vi "Rational Resample (single channel, CDB).vi"(5 "anti-aliasing?":bool=TRUE, 6 "FIR filter specifications":T1={"alias rejection (dB)"=120.0, "normalized bandwidth"=0.4536} {"normalized bandwidth" format="%.4f"; "alias rejection (dB)" format="%.2f"}, 7 "reset":bool, 8 "error in (no error)":errorcluster, 9 "resample factor":cluster{"interpolation":i32, "decimation":i32}={"interpolation"=1, "decimation"=1}, 10 "start index":i32, 11 "X":cdb[](array[numeric])) -> (0 "error out":errorcluster, 2 "t0":dbl, 3 "Y":cdb[](array[numeric]))   [LabVIEW 2014, in "NI_AALPro.lvlib"]
doc: "Resamples the input signal <B>X</B> by interpolating <B>X</B>, passing the interpolated signal through an FIR filter, and decimating the filtered signal. Wire data to the <B>X</B> input to determine the polymorphic instance to use or manually select the instance."
uses:
  NI_AALPro.lvlib
  lvanlys.dll
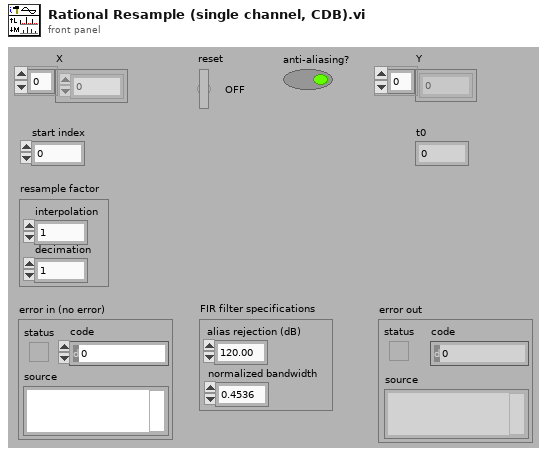
[diagram p1: front panel]
types:
  T1 = cluster{"alias rejection (dB)":dbl, "normalized bandwidth":dbl}
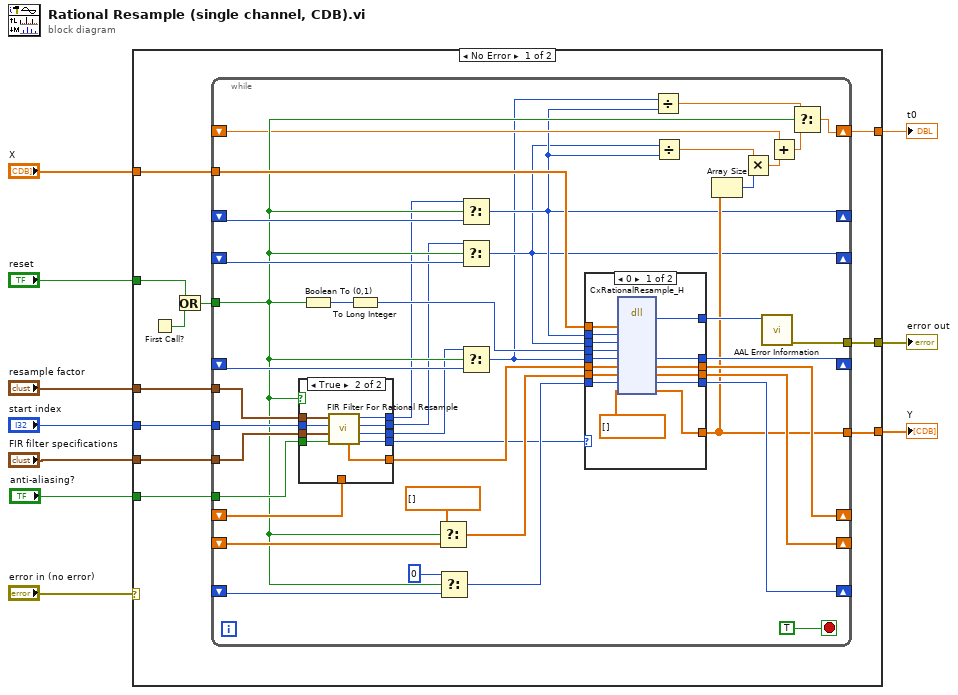
[diagram p0: block diagram]
diagram:
  n1 = case shown="No Error" "error in (no error)" {
    selector: "error in (no error)" -> [_ w89]
    tunnel: "X" -> [w21 _]
    tunnel: "FIR filter specifications" -> [w20 _]
    tunnel: "start index" -> [w19 _]
    tunnel: [w18 w89] -> w7
    tunnel: "resample factor" -> [w17 _]
    tunnel: [w16 _] -> w5
    tunnel: "anti-aliasing?" -> [w15 _]
    tunnel: [w14 _] -> w2
    tunnel: "reset" -> [w11 _]
    frame No Error {
      n2 = First Call?() -> (First Call?: T/F=w13:bool)
      n3 = Or(x=w11, y=w13) -> (x .or. y?=w12:bool)
      n4 = while {
        tunnel: w21 -> [w62]
        shift-right: [w25] -> _
        shift-left: _ -> [w60]
        tunnel: w12 -> [w36]
        shift-right: [w24] -> _
        shift-left: _ -> [w59]
        shift-right: [w43] -> _
        shift-left: _ -> [w56]
        shift-right: [w44] -> _
        shift-left: _ -> [w54]
        shift-right: [w50] -> _
        shift-left: _ -> [w51]
        shift-right: [w47] -> _
        shift-left: _ -> [w46]
        tunnel: w20 -> [w49]
        tunnel: w19 -> [w45]
        tunnel: [w41] -> w18
        tunnel: w17 -> [w40]
        tunnel: [w33] -> w16
        tunnel: w15 -> [w37]
        shift-right: [w34] -> w14
        shift-left: _ -> [w27]
        stop <- TRUE stop-if-true
        n5 = case shown="True" w36 {
          tunnel: [w79 w82] -> w48
          tunnel: w49 -> [_ w83]
          tunnel: w46 -> [w79 _]
          tunnel: [_ w88] -> w32
          tunnel: [_ w87] -> w31
          tunnel: w45 -> [_ w84]
          tunnel: [_ w86] -> w22
          tunnel: w40 -> [_ w85]
          tunnel: [_ w81] -> w39
          tunnel: w37 -> [_ w80]
          frame False {
          }
          frame True {
            n6 = call "FIR Filter For Rational Resample.vi"("anti-aliasing?"=w80, "FIR filter specifications"=w83, "start index"=w84, "resample factor"=w85) -> ("error"=w81:i32, "start index out"=w86:i32, "decimation"=w87:i32, "interpolation out"=w88:i32, "filter coefficients"=w82:dbl[])  [unwired: 3 in]
          }
        }
        n7 = Boolean To (0,1)(Boolean=w36) -> (0, 1=w58:i16)
        n8 = To Long Integer(number=w58) -> (32bit integer=w57:i32)
        n9 = Select(t=cdb[] [] ("yH"), s=w36, f=w56) -> (s? t:f=w52:cdb[])
        n10 = Select(t=0, s=w36, f=w54) -> (s? t:f=w53:i32)
        n11 = Select(t=w32, s=w36, f=w60) -> (s? t:f=w25:i32)
        n12 = Select(t=w31, s=w36, f=w59) -> (s? t:f=w24:i32)
        n13 = Select(t=w22, s=w36, f=w51) -> (s? t:f=w23:i32)
        n14 = case shown="0" w39 {
          selector: w39 -> [_ w78]
          tunnel: w62 -> [w77 _]
          tunnel: w25 -> [w76 _]
          tunnel: w24 -> [w75 _]
          tunnel: w57 -> [w74 _]
          tunnel: w53 -> [w73 _]
          tunnel: w52 -> [w66 _]
          tunnel: w23 -> [w72 _]
          tunnel: [w71 _] -> w50
          tunnel: w48 -> [w70 _]
          tunnel: [w69 _] -> w47
          tunnel: [w68 _] -> w44
          tunnel: [w65 _] -> w43
          tunnel: [w67 w78] -> w42
          tunnel: [w63 _] -> w33
          frame 0 {
            n15 = dll-call lib="C:/Program Files (x86)/National Instruments/LabVIEW 2014/resource/lvanlys.*" fn="CxRationalResample_H"("X"=w77, "interpolation"=w76, "decimation"=w75, "reset"=w74, "startIndex"=w72, "filterH"=w70, "yH"=w66, "singalSizeInBuffer"=w73, "yH"=cdb[] []) -> (w67:i32, "startIndex"=w71:i32, "filterH"=w69:dbl[], "yH"=w65:cdb[], "singalSizeInBuffer"=w68:i32, "yH"=w63:cdb[])  [unwired: 7 in, 2 out]
          }
          frame 1, Default {
          }
        }
        n16 = Divide(x=w23, y=w25) -> (x/y=w35:dbl)
        n17 = Divide(x=w24, y=w25) -> (x/y=w29:dbl)
        n18 = Array Size(array=w33) -> (size(s)=w30:i32)
        n19 = Multiply(x=w29, y=w30) -> (x*y=w28:dbl)
        n20 = call "AAL Error Information.vi"("error code"=w42) -> ("error out"=w41:errorcluster)  [unwired: 10 in]
        n21 = Add(x=w27, y=w28) -> (x+y=w26:dbl)
        n22 = Select(t=w35, s=w36, f=w26) -> (s? t:f=w34:dbl)
      }
    }
    frame Error {
    }
  }
  "error out" <- w7
  "Y" <- w5
  "t0" <- w2
